vi "Measurement Logic.vi"() -> ()   [LabVIEW 2021, in "ImageRendering.lvlib"]
uses:
  ImageRendering.lvlib
  Measurement Configuration.ctl
  Measurement Results.ctl
  <vilib>/MeasurementLink/MeasurementLink Measurement Server/Measure Call Context/Measure Call Context.lvclass
panel:
  out "Image":T1(plugin-control)
  out "measure call context out":refnum<class "Measure Call Context.lvclass">
  in  "measure call context in":refnum<class "Measure Call Context.lvclass">
  out "measurement results":T2={"Image Data"="Empty", "File Size (MB)"=0.0, "Image Pixels (U32)"=[], "Image Acq time"=""}
  in  "measurement configuration":T3={"Image Path"="D:\\Avi\\_PRK5307.jpg", "Image Converison Type"=""}
  out "error out":errorcluster
  in  "error in":errorcluster
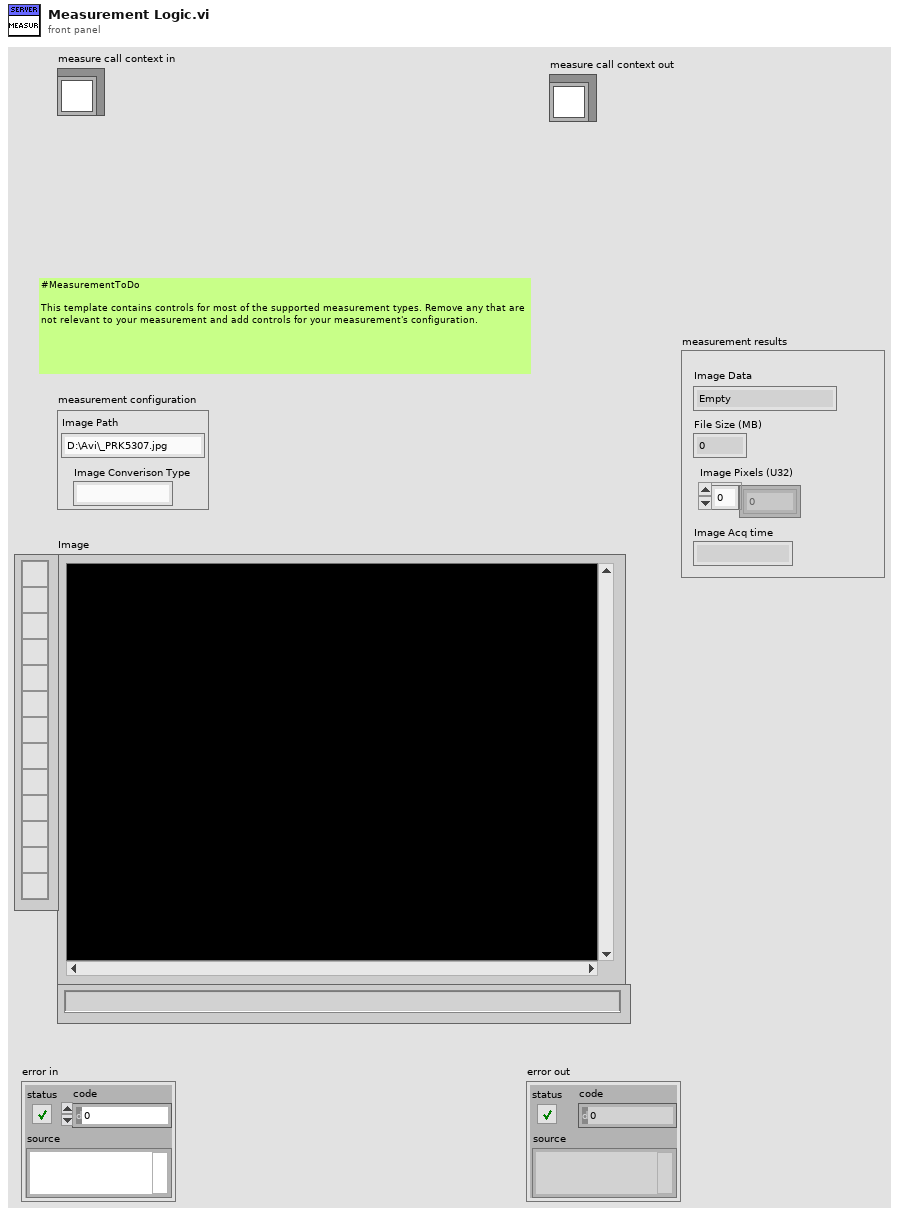
[diagram p1: front panel]
types:
  T1 = typedef "IMAQ Image.ctl" = refnum<image>
  T2 = typedef "ImageRendering.lvlib/Measurement Results.ctl" = cluster{"Image Data":string, "File Size (MB)":dbl, "Image Pixels (U32)":u32[], "Image Acq time":string}
  T3 = typedef "ImageRendering.lvlib/Measurement Configuration.ctl" = cluster{"Image Path":string, "Image Converison Type":string}
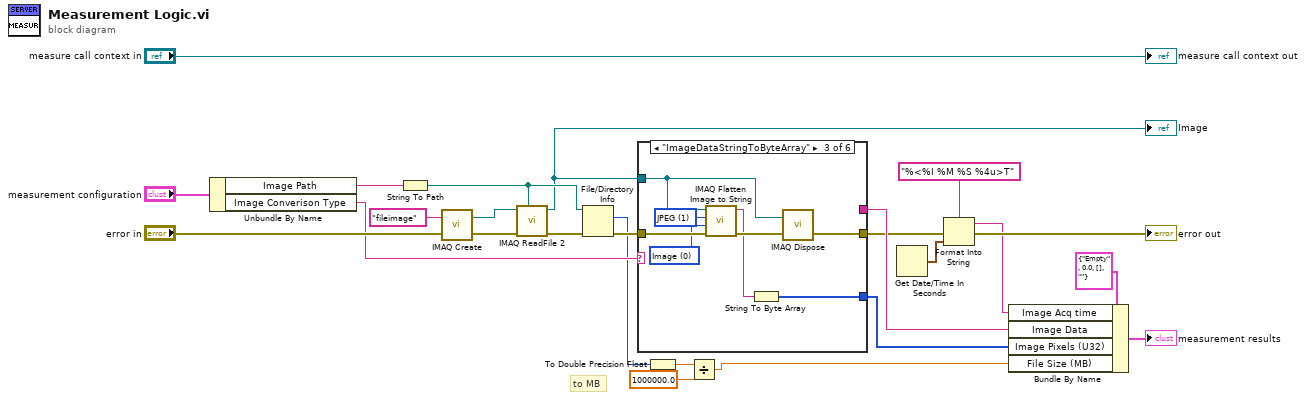
[diagram p0: block diagram]
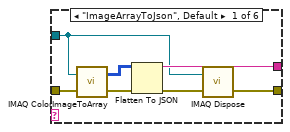
[diagram p2: hidden frame]
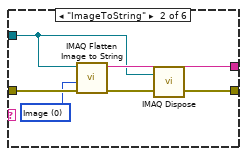
[diagram p3: hidden frame]
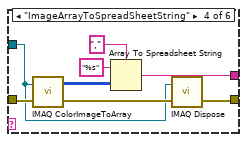
[diagram p4: hidden frame]
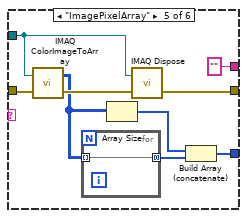
[diagram p5: hidden frame]
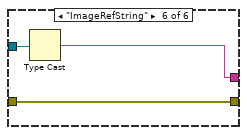
[diagram p6: hidden frame]
diagram:
  # "to MB"
  n1 = Unbundle By Name("measurement configuration") -> ("Image Path"=w21:string, "Image Converison Type"=w13:string)
  n2 = String To Path(string=w21) -> (path=w16:path)
  n3 = call "IMAQ Create"("Image Name"="fileimage", "error in (no error)"="error in") -> ("New Image"=w19:T1, "error out"=w18:errorcluster)  [unwired: 3 in]
  n4 = call "IMAQ ReadFile 2"("File Path"=w16, "error in (no error)"=w18, "Image"=w19) -> ("error out"=w15:errorcluster, "Image Out"=w12:T1)  [unwired: 4 in, 3 out]
  "Image" <- w12
  n5 = File/Directory Info(path=w16, error in=w15) -> (size=w4:i64, error out=w14:errorcluster)  [unwired: 5 out]
  n6 = case shown="\"ImageDataStringToByteArray\"" w13 {
    tunnel: w14 -> [w32 w38 w46 w54 w63 w67]
    tunnel: [w27 w34 w43 w48 w56 w67] -> w7
    tunnel: [w29 w36 _ w50 "" ("spreadsheet string") w65] -> w11
    tunnel: w12 -> [w26 w33 w42 w47 w55 w66]
    tunnel: [_ _ w39 _ w58 _] -> w10
    frame "ImageArrayToJson", Default {
      n7 = call "IMAQ ColorImageToArray"("Image"=w26, "error in (no error)"=w32) -> ("Image Pixels (U32)"=w28:u32[][], "error out"=w31:errorcluster)  [unwired: 2 in, 1 out]
      n8 = Flatten To JSON(anything=w28, error in (no error)=w31) -> (JSON string=w29:string, 11:w30:errorcluster)  [unwired: 1 in]
      n9 = call "IMAQ Dispose"("Image"=w26, "error in (no error)"=w30) -> ("error out"=w27:errorcluster)  [unwired: 4 in]
    }
    frame "ImageToString" {
      w35 = 0 items=["Image", "Image and Vision Info", "Reference to Image"] ("Type of Flatten (Image and Vision Info)")
      n10 = call "IMAQ Flatten Image to String"("error in (no error)"=w38, "Type of Flatten (Image and Vision Info)"=w35, "Image"=w33) -> ("error out"=w37:errorcluster, "Data String"=w36:string)  [unwired: 7 in]
      n11 = call "IMAQ Dispose"("Image"=w33, "error in (no error)"=w37) -> ("error out"=w34:errorcluster)  [unwired: 4 in]
    }
    frame "ImageDataStringToByteArray" {
      w41 = 1 items=["None", "JPEG", "PACKED BINARY"] ("Compression (None)")
      w44 = 0 items=["Image", "Image and Vision Info", "Reference to Image"] ("Type of Flatten (Image and Vision Info)")
      n12 = call "IMAQ Flatten Image to String"("error in (no error)"=w46, "Type of Flatten (Image and Vision Info)"=w44, "Compression (None)"=w41, "Image"=w42) -> ("error out"=w45:errorcluster, "Data String"=w40:string)  [unwired: 6 in]
      n13 = String To Byte Array(string=w40) -> (unsigned byte array=w39:u8[])
      n14 = call "IMAQ Dispose"("Image"=w42, "error in (no error)"=w45) -> ("error out"=w43:errorcluster)  [unwired: 4 in]
    }
    frame "ImageArrayToSpreadSheetString" {
      n15 = call "IMAQ ColorImageToArray"("Image"=w47, "error in (no error)"=w54) -> ("Image Pixels (U32)"=w52:u32[][], "error out"=w53:errorcluster)  [unwired: 2 in, 1 out]
      n16 = Array To Spreadsheet String(delimiter (Tab)=",", array=w52, 3:"%s" ("format string")) -> (spreadsheet string=w50:string)
      n17 = call "IMAQ Dispose"("Image"=w47, "error in (no error)"=w53) -> ("error out"=w48:errorcluster)  [unwired: 4 in]
    }
    frame "ImagePixelArray" {
      n18 = call "IMAQ ColorImageToArray"("Image"=w55, "error in (no error)"=w63) -> ("Image Pixels (U32)"=w61:u32[][], "error out"=w62:errorcluster)  [unwired: 2 in, 1 out]
      n19 = for {
        tunnel: w61 -> [w64] mode=indexing
        tunnel: [w64] -> w59 mode=concatenating
      }
      n20 = Array Size(array=w61) -> (size(s)=w60:i32[])
      n21 = call "IMAQ Dispose"("Image"=w55, "error in (no error)"=w62) -> ("error out"=w56:errorcluster)  [unwired: 4 in]
      n22 = Build Array (concatenate)(w60, w59) -> (w58:u32[])
    }
    frame "ImageRefString" {
      n23 = Type Cast(x=w66) -> (*(type *) &x=w65:string)  [unwired: 1 in]
    }
  }
  n24 = To Double Precision Float(number=w4) -> (double precision float=w3:dbl)
  n25 = Divide(x=w3, y=1000000.0) -> (x/y=w1:dbl)
  n26 = Get Date/Time In Seconds() -> (seconds since 1Jan1904=w8:timestamp)
  n27 = Format Into String(format string="%<%I %M %S %4u>T", error in=w7, w8) -> (resulting string=w5:string, error out=→"error out":errorcluster)  [unwired: 1 in]
  n28 = Bundle By Name(cluster=T2 {"Image Data"="Empty", "File Size (MB)"=0.0, "Image Pixels (U32)"=[], "Image Acq time"=""} ("Measurement Results"), "Image Acq time"=w5, "Image Data"=w11, "Image Pixels (U32)"=w10, "File Size (MB)"=w1) -> (→"measurement results":T2)
  "measure call context out" <- "measure call context in"
